vi "HW Config.vi"(8 "error in (no error)":errorcluster, 11 "start path":path=path "") -> (0 "error out":errorcluster, 2 "HW config 2":T1={"DMM"="COM15", "mux"="COM11", "demux"="COM16", "eMIC1"="COM13", "eMIC2"="COM6", "eMIC3"="COM9", "eMIC4"="COM10", "eMIC5"="COM12", "eMIC6"="COM11"})   [LabVIEW 2018, in "Application.lvlib"]
uses:
  Application.lvlib
  type defs/HW config.ctl
  <vilib>/Utility/config.llb/Read Key (String).vi
  <vilib>/Utility/config.llb/NI_LVConfig.lvlib
panel:
  in  "HW config":T1={"DMM"="COM15", "mux"="COM11", "demux"="COM16", "eMIC1"="COM16", "eMIC2"="COM16", "eMIC3"="COM16", "eMIC4"="COM16", "eMIC5"="COM16", "eMIC6"="COM16"}
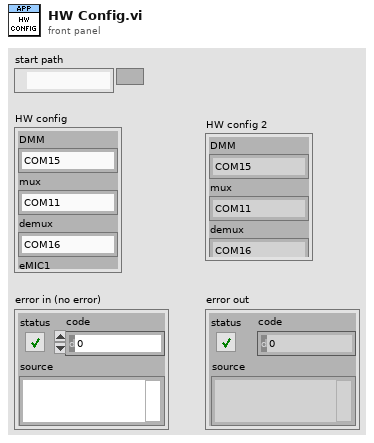
[diagram p1: front panel]
types:
  T1 = typedef "Application.lvlib/HW config.ctl" = cluster{"DMM":string, "mux":string, "demux":string, "eMIC1":string, "eMIC2":string, "eMIC3":string, "eMIC4":string, "eMIC5":string, "eMIC6":string}
  T2 = typedef "NI_LVConfig.lvlib/Config Data RefNum.ctl" = refnum<k1>
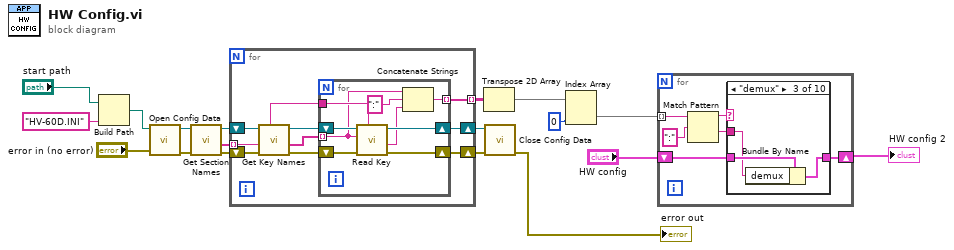
[diagram p0: block diagram]
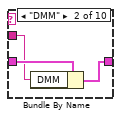
[diagram p3: hidden frame]
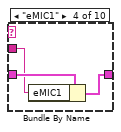
[diagram p4: hidden frame]
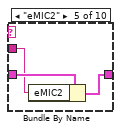
[diagram p5: hidden frame]
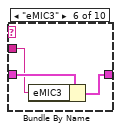
[diagram p6: hidden frame]
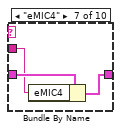
[diagram p7: hidden frame]
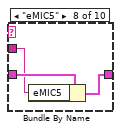
[diagram p8: hidden frame]
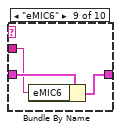
[diagram p9: hidden frame]
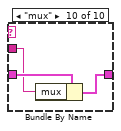
[diagram p10: hidden frame]
diagram:
  n1 = Build Path(base path="start path", name or relative path="HV-60D.INI") -> (appended path=w3:path)
  n2 = call <vilib>:"Open Config Data.vi"("error in (no error)"="error in (no error)", "configuration file path"=w3) -> ("error out"=w11:errorcluster, "refnum"=w12:T2)  [unwired: 7 in, 1 out]
  n3 = call <vilib>:"Get Section Names.vi"("error in (no error)"=w11, "refnum"=w12) -> ("error out"=w16:errorcluster, "section names"=w18:string[], "refnum out"=w17:T2)  [unwired: 7 in]
  n4 = for {
    tunnel: w18 -> [w19] mode=indexing
    shift-right: [w23] -> w15
    shift-left: w17 -> [w27]
    tunnel: [w24] -> w13 mode=indexing
    shift-right: [w20] -> w14
    shift-left: w16 -> [w21]
    n5 = call <vilib>:"Get Key Names.vi"("section"=w19, "error in (no error)"=w21, "refnum"=w27) -> ("error out"=w22:errorcluster, "key names"=w26:string[], "refnum out"=w25:T2)  [unwired: 5 in, 1 out]
    n6 = for {
      tunnel: w26 -> [w31] mode=indexing
      shift-right: [w35] -> w23
      shift-left: w25 -> [w36]
      tunnel: w19 -> [w34]
      tunnel: [w28] -> w24 mode=indexing
      shift-right: [w33] -> w20
      shift-left: w22 -> [w32]
      n7 = call-poly <vilib>:"Read Key.vi"("section"=w34, "error in (no error)"=w32, "key"=w31, "refnum"=w36) -> ("error out"=w33:errorcluster, "value"=w30:string, "refnum out"=w35:T2)  [unwired: 4 in, 1 out]
      n8 = Concatenate Strings(w31, ":" ("string"), w30) -> (w28:string)
    }
  }
  n9 = Transpose 2D Array(2D array=w13) -> (transposed array=w10:string[][])
  n10 = call <vilib>:"Close Config Data.vi"("error in (no error)"=w14, "refnum"=w15) -> ("error out"=→"error out":errorcluster)  [unwired: 8 in, 1 out]
  n11 = Index Array(array=w10, index (col)=0 ("disabled index (col)")) -> (element=w8:string[])  [unwired: 1 in]
  n12 = for {
    tunnel: w8 -> [w41] mode=indexing
    shift-right: [w37] -> w6
    shift-left: "HW config" -> [w39]
    n13 = Match Pattern(string=w41, regular expression=":") -> (before substring=w40:string, after substring=w38:string)  [unwired: 1 in, 2 out]
    n14 = case shown="\"demux\"" w40 {
      tunnel: w39 -> [w43 w46 w49 w52 w55 w58 w61 w64 w67 w70]
      tunnel: w38 -> [_ w45 w48 w51 w54 w57 w60 w63 w65 w69]
      tunnel: [w43 w44 w47 w50 w53 w56 w59 w62 w66 w68] -> w37
      frame "False", Default {
      }
      frame "DMM" {
        n15 = Bundle By Name(cluster=w46, "DMM"=w45) -> (w44:T1)
      }
      frame "demux" {
        n16 = Bundle By Name(cluster=w49, "demux"=w48) -> (w47:T1)
      }
      frame "eMIC1" {
        n17 = Bundle By Name(cluster=w52, "eMIC1"=w51) -> (w50:T1)
      }
      frame "eMIC2" {
        n18 = Bundle By Name(cluster=w55, "eMIC2"=w54) -> (w53:T1)
      }
      frame "eMIC3" {
        n19 = Bundle By Name(cluster=w58, "eMIC3"=w57) -> (w56:T1)
      }
      frame "eMIC4" {
        n20 = Bundle By Name(cluster=w61, "eMIC4"=w60) -> (w59:T1)
      }
      frame "eMIC5" {
        n21 = Bundle By Name(cluster=w64, "eMIC5"=w63) -> (w62:T1)
      }
      frame "eMIC6" {
        n22 = Bundle By Name(cluster=w67, "eMIC6"=w65) -> (w66:T1)
      }
      frame "mux" {
        n23 = Bundle By Name(cluster=w70, "mux"=w69) -> (w68:T1)
      }
    }
  }
  "HW config 2" <- w6
